vi "Function.vi"(8 "error in (no error)":errorcluster, 9 "Numeric B":cxt, 10 "Numeric A":cxt, 11 "Two Terminal in":refnum<class "Greater_CPLX_EXT.lvclass">) -> (0 "error out":errorcluster, 2 "Result":bool, 3 "Two Terminal out":refnum<class "Greater_CPLX_EXT.lvclass">)   [LabVIEW 2021, in "Greater_CPLX_EXT.lvclass"]
uses:
  Greater_CPLX_EXT.lvclass
  Greater_CPLX_EXT.lvclass/Greater_CPLX_EXT.ctl
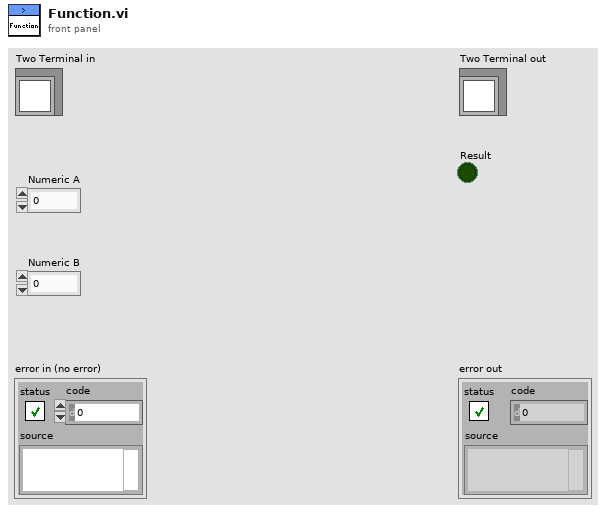
[diagram p1: front panel]
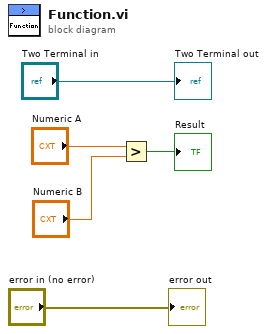
[diagram p0: block diagram]
diagram:
  n1 = Greater?(x="Numeric A", y="Numeric B") -> (0:→"Result":bool)
  "error out" <- "error in (no error)"
  "Two Terminal out" <- "Two Terminal in"
